vi "LED Configure.vi"(8 "LED On":bool, 10 "Refnum Name":string="UseGlobal", 11 "LEDChannel":T1) -> ()   [LabVIEW 2019]
uses:
  Globals/LED_Globals.vi
  <vilib>/Rock Robotics/WPI/ThirdParty/Phoenix-LabVIEW/CANifier/CTRE_CANifier_LEDChannel.ctl
panel:
  # "This VI turns a single \nLED channel on."
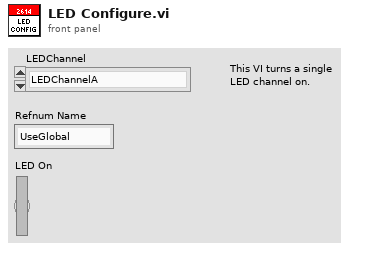
[diagram p1: front panel]
types:
  T1 = typedef "CTRE_CANifier_LEDChannel.ctl" = enum32{"LEDChannelA", "LEDChannelB", "LEDChannelC"}
  T2 = typedef "CTRE_CANifier_DeviceRef.ctl" = cluster{"DeviceStatus":errorcluster, "Device Number":u8, "Handle":u64, "UsageFrame":u32, "Library Path":path}
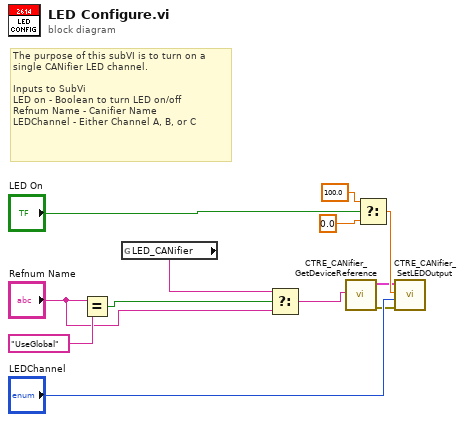
[diagram p0: block diagram]
diagram:
  # "The purpose of this subVI is to turn on a single CANifier LED channel.\n\nInputs to SubVi\nLED on - Boolean to turn LED on/off\nRefnum Name - Canifier Name\nLEDChannel - Either Channel A, B, or C"
  n1 = Equal?(x="Refnum Name", y="UseGlobal") -> (x = y?=w2:bool)
  n2 = global read "LED_Globals.vi" "LED_CANifier"() -> (w6:string)
  n3 = Select(t=w6, s=w2, f="Refnum Name") -> (s? t:f=w5:string)
  n4 = call <vilib>:"CTRE_CANifier_GetDeviceReference.vi"("refnum name"=w5) -> ("error out"=w8:errorcluster, "CANifierDevRef"=w7:T2)  [unwired: 9 in]
  n5 = Select(t=100.0, s="LED On", f=0.0) -> (s? t:f=w12:dbl)
  n6 = call <vilib>:"CTRE_CANifier_SetLEDOutput.vi"("error in"=w8, "LEDChannel"="LEDChannel", "Percent Output"=w12, "CANifierDevRef"=w7) -> ()  [unwired: 6 in, 2 out]
